vi "CM-Get Digital Lines.vi"(0 "Path In":path, 2 "Section":T1=enum."Digital Inputs", 11 "error in (no error)":errorcluster) -> (4 "Path Out":path, 6 "Endpoints":string[](array[string]), 10 "Lines":i32[](array[numeric]), 15 "error out":errorcluster)   [LabVIEW 2020]
uses:
  Type Defs/CM-IO Type.ctl
  <vilib>/Utility/config.llb/Read Key (String).vi
  <vilib>/Utility/config.llb/NI_LVConfig.lvlib
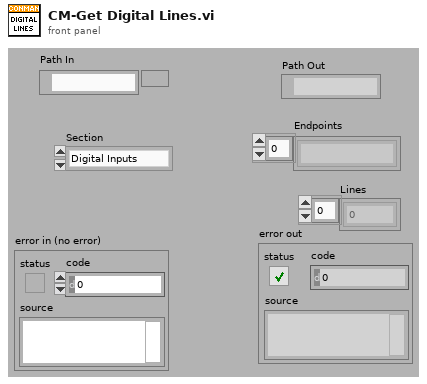
[diagram p1: front panel]
types:
  T1 = typedef "CM-IO Type.ctl" = enum16{"Analog Outputs", "Analog Inputs", "Digital Outputs", "Digital Inputs"}
  T2 = typedef "NI_LVConfig.lvlib/Config Data RefNum.ctl" = refnum<k1>
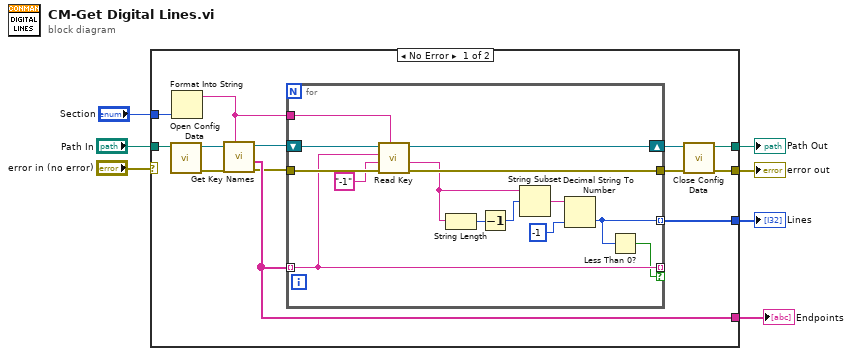
[diagram p0: block diagram]
diagram:
  n1 = case shown="No Error" "error in (no error)" {
    selector: "error in (no error)" -> [_ w36]
    tunnel: [w20 w35] -> w7
    tunnel: [w17 w36] -> w6
    tunnel: "Path In" -> [w16 w35]
    tunnel: [w13 _] -> w3
    tunnel: [w10 _] -> w2
    tunnel: "Section" -> [w9 _]
    frame No Error {
      n2 = call <vilib>:"Open Config Data.vi"("configuration file path"=w16) -> ("error out"=w15:errorcluster, "refnum"=w14:T2)  [unwired: 8 in, 1 out]
      n3 = Format Into String(w9) -> (resulting string=w8:string)  [unwired: 3 in, 1 out]
      n4 = call <vilib>:"Get Key Names.vi"("section"=w8, "error in (no error)"=w15, "refnum"=w14) -> ("error out"=w11:errorcluster, "key names"=w13:string[], "refnum out"=w12:T2)  [unwired: 5 in, 1 out]
      n5 = for {
        tunnel: w11 -> [w33]
        tunnel: w13 -> [w23] mode=indexing
        tunnel: [w30] -> w18
        shift-right: [w31] -> w19
        shift-left: w12 -> [w34]
        tunnel: [w24] -> w10 mode=indexing
        tunnel: [w23] -> _ mode=indexing if=w22
        tunnel: w8 -> [w21]
        n6 = call-poly <vilib>:"Read Key.vi"("section"=w21, "error in (no error)"=w33, "default value"="-1", "key"=w23, "refnum"=w34) -> ("error out"=w30:errorcluster, "value"=w29:string, "refnum out"=w31:T2)  [unwired: 3 in, 1 out]
        n7 = String Length(string=w29) -> (length=w28:i32)
        n8 = Decrement(x=w28) -> (x-1=w27:i32)
        n9 = String Subset(string=w29, offset (0)=w27) -> (substring=w26:string)  [unwired: 1 in]
        n10 = Decimal String To Number(string=w26, default (0L)=-1 ("default (0 I32)")) -> (number=w24:i32)  [unwired: 1 in, 1 out]
        n11 = Less Than 0?(x=w24) -> (x < 0?=w22:bool)
      }
      n12 = call <vilib>:"Close Config Data.vi"("error in (no error)"=w18, "refnum"=w19) -> ("error out"=w17:errorcluster, "file path"=w20:path)  [unwired: 8 in]
    }
    frame Error {
    }
  }
  "error out" <- w6
  "Path Out" <- w7
  "Lines" <- w2
  "Endpoints" <- w3
